vi "Create Repeated Peak Ramp.vi"(0 "P1 Peak Array":dbl[](array[numeric]), 5 "Start":dbl, 7 "Step":dbl, 11 "Error In":errorcluster) -> (4 "Array 2":dbl[](array[numeric]), 15 "Error Out":errorcluster)   [LabVIEW 2013]
uses:
  <vilib>/Analysis/1siggen.llb/Ramp Pattern by Delta.vi
  <vilib>/Analysis/NI_AALBase.lvlib
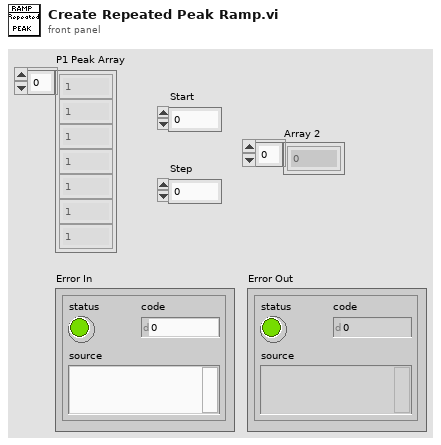
[diagram p1: front panel]
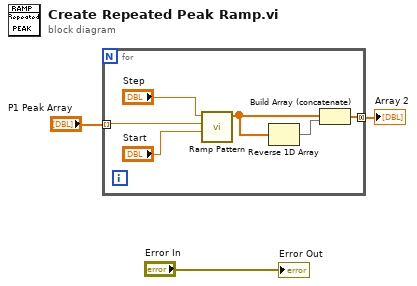
[diagram p0: block diagram]
diagram:
  n1 = for {
    tunnel: "P1 Peak Array" -> [w7] mode=indexing
    tunnel: [w6] -> w2 mode=concatenating
    n2 = call-poly <vilib>:"Ramp Pattern.vi"("start"="Start", "end"=w7, "delta"="Step") -> ("Ramp Pattern"=w5:dbl[])  [unwired: 6 in, 2 out]
    n3 = Reverse 1D Array(array=w5) -> (reversed array=w4:dbl[])
    n4 = Build Array (concatenate)(w5, w4) -> (w6:dbl[])
  }
  "Array 2" <- w2
  "Error Out" <- "Error In"
